vi "Advance past next JSON Scaler.vi"(7 "JSON":string, 9 "Offset":i32, 11 "Parser State in":T1=enum."Leading Whitespace") -> (1 "Offset Past":i32, 3 "Parser State":T1=enum."Value end", 6 "Value start":i32)   [LabVIEW 2017, in "JSONtext.lvlib"]
uses:
  JSONtext.lvlib
  Parsing State.ctl
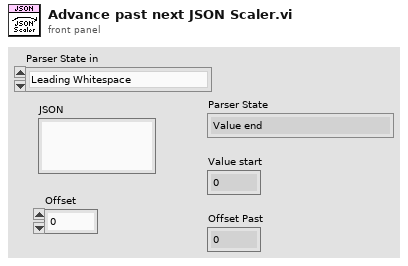
[diagram p1: front panel]
types:
  T1 = typedef "JSONtext.lvlib/Parsing State.ctl" = enum16{"Parser Error", "Object", "Array", "String", "Number/Other", "Leading Whitespace", "Object end", "Array end", "Value end"}
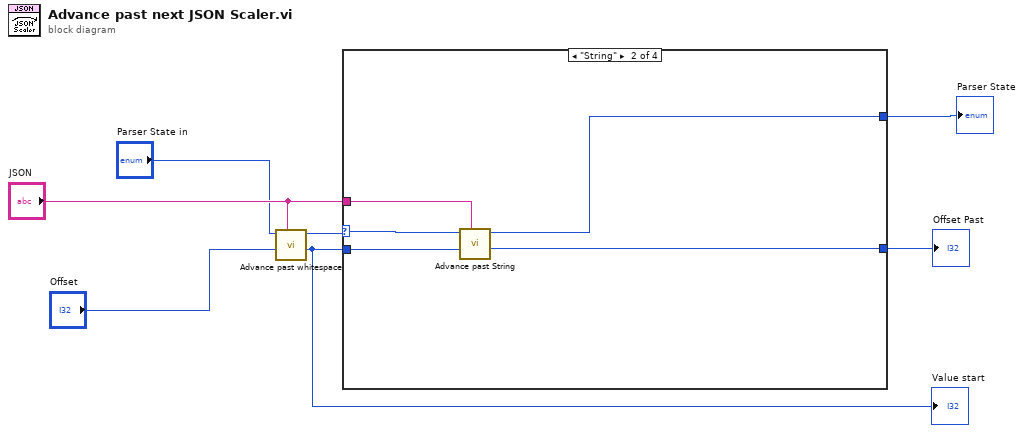
[diagram p0: block diagram]
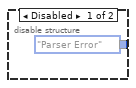
[diagram p3: hidden frame]
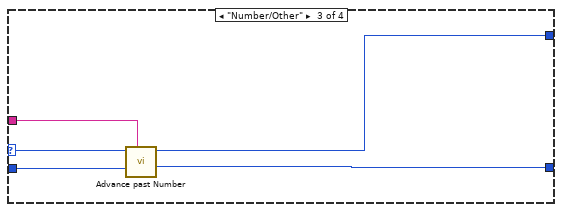
[diagram p4: hidden frame]
diagram:
  n1 = call "Advance past whitespace.vi"("JSON"="JSON", "Offset"="Offset", "Parser State in"="Parser State in") -> ("Offset of first non-whitespace"=w2:i32, "Parser State"=w6:T1)  [unwired: 7 in]
  "Value start" <- w2
  n2 = case shown="\"String\"" w6 {
    selector: w6 -> [w8 w16 w21 w24]
    tunnel: "JSON" -> [_ w17 w22 _]
    tunnel: w2 -> [w10 w15 w20 w23]
    tunnel: [w10 w14 w19 w23] -> w5
    tunnel: [w9 w13 w18 w24] -> w4
    frame "Parser Error", Default {
      n3 = disable-structure shown="Enabled" {
        disable-tunnel: [Parsing_State."Parser Error" ("State") w12] -> w9
        disable-tunnel: w8 -> [_ w12]
        frame Disabled {
        }
        frame Enabled {
        }
      }
    }
    frame "String" {
      n4 = call "Advance past String.vi"("JSON"=w17, "Offset"=w15, "State in"=w16) -> ("Offset past match"=w14:i32, "State"=w13:T1)  [unwired: 6 in, 1 out]
    }
    frame "Number/Other" {
      n5 = call "Advance past Number.vi"("JSON"=w22, "Offset (0)"=w20, "Parser State in"=w21) -> ("Offset past match"=w19:i32, "Parser State"=w18:T1)  [unwired: 5 in, 2 out]
    }
    frame "Object", "Array" {
      # "Note that big JSON text will have lots of scalers compared to Objects/Arrays"
      # "This VI is inlined, for speed.  We cannot inline anything in a recursive cycle\nso we can't do Arrays/Objects here (must call a non-inlined VI after)"
    }
  }
  "Parser State" <- w4
  "Offset Past" <- w5
